vi "GetAttribute.vi"(8 "error in (no error)":errorcluster, 11 "Data_General in":refnum<class "Data_FrameInfo.lvclass">) -> (0 "error out":errorcluster, 2 "Attribute":T1, 3 "Data_General out":refnum<class "Data_FrameInfo.lvclass">)   [LabVIEW 2020, in "Data_FrameInfo.lvclass"]
uses:
  Data_FrameInfo.lvclass
  Attribute.vi
  Data_FrameInfo.lvclass/Data_FrameInfo.ctl
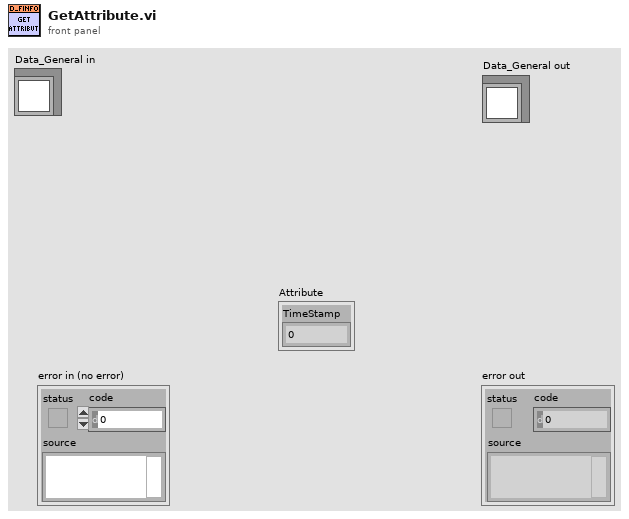
[diagram p1: front panel]
types:
  T1 = typedef "Data_FrameInfo.lvclass/Attribute.vi" = cluster{"TimeStamp":u64}
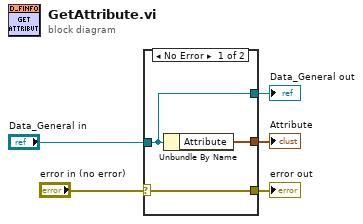
[diagram p0: block diagram]
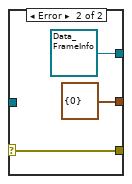
[diagram p2: hidden frame]
diagram:
  n1 = case shown="No Error" "error in (no error)" {
    selector: "error in (no error)" -> [w8 w11]
    tunnel: [w8 w11] -> w4
    tunnel: [w7 refnum<class "Data_FrameInfo.lvclass"> refnum ("Data_Pupil_Diameter in")] -> w3
    tunnel: "Data_General in" -> [w7 _]
    tunnel: [w6 T1 {"TimeStamp"=0} ("Attribute")] -> w1
    frame No Error {
      n2 = Unbundle By Name(w7) -> ("Attribute"=w6:T1)
    }
    frame Error {
    }
  }
  "error out" <- w4
  "Data_General out" <- w3
  "Attribute" <- w1
